vi "Receive Monitoring Frame.vi"(11 "Test Case In":refnum<class "Test HSU MCU V2.lvclass">) -> (0 "error out":errorcluster, 3 "Test Case Out":refnum<class "Test HSU MCU V2.lvclass">)   [LabVIEW 2024, in "Test HSU MCU V2.lvclass"]
uses:
  Test HSU MCU V2.lvclass
  C:/Program Files/National Instruments/LabVIEW 2024/vi.lib/Astemes/LUnit/Test Case.lvclass
  HSU MCU V2 CFG/HSU MCU V2 CFG.lvclass
  D:/git/HAL/HAL/Configurations/CFG JSON/CFG JSON.lvclass
  <vilib>/Astemes/LUnit/Test Case.lvclass/Test Case.ctl
  <vilib>/Astemes/LUnit/Append Pass Result.vi
  <vilib>/Astemes/LUnit/Append Fail Result.vi
  <vilib>/Astemes/LUnit/Run In UI.vi
  <vilib>/Utility/error.llb/Clear Errors.vi
  <vilib>/Astemes/LUnit/Test Case.lvclass
  Configurations/CFG JSON/CFG JSON.lvclass
panel:
  out "Output":variant
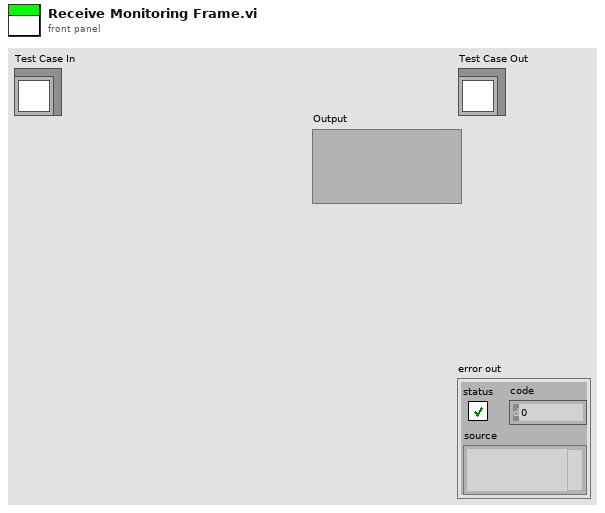
[diagram p1: front panel]
types:
  T1 = cluster{"Action":enum16{"Read", "Write"}, "Point Ident":string, "Data":variant}
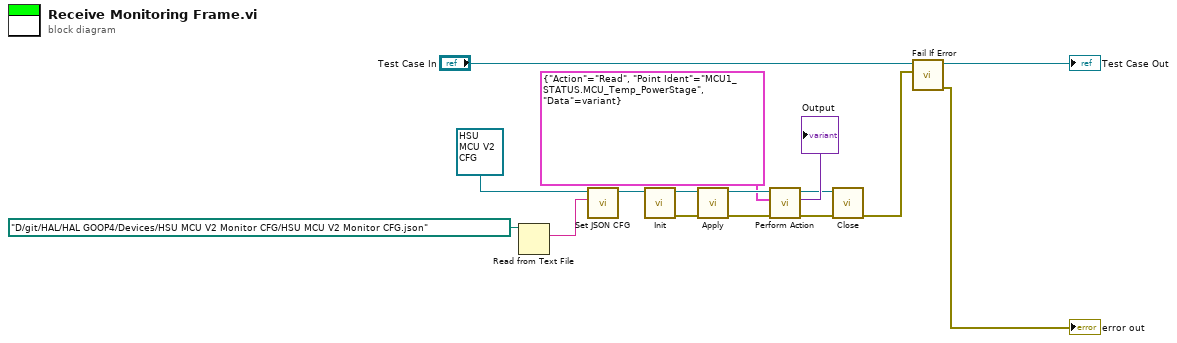
[diagram p0: block diagram]
diagram:
  n1 = Read from Text File(file (use dialog)=path "D:/git/HAL/HAL GOOP4/Devices/HSU MCU V2 Monitor CFG/HSU MCU V2 Monitor CFG.json") -> (text=w4:string)  [unwired: 3 in, 3 out]
  n2 = call "Set JSON CFG.vi"("<JSON> CFG"=w4, "CFG JSON in"=refnum<class "HSU MCU V2 CFG.lvclass"> refnum ("CFG Base in")) -> ("CFG JSON out"=w12:refnum<class "HSU MCU V2 CFG.lvclass">)  [unwired: 9 in]
  n3 = call-dynamic "Init.vi"("CFG Base in"=w12) -> ("error out"=w11:errorcluster, "CFG Base out"=w10:refnum<class "HSU MCU V2 CFG.lvclass">)  [unwired: 9 in]
  n4 = call-dynamic "Apply.vi"("error in"=w11, "HSU MCU V2 in"=w10) -> ("error out"=w9:errorcluster, "HSU MCU V2 out"=w8:refnum<class "HSU MCU V2 CFG.lvclass">)  [unwired: 8 in]
  n5 = call-dynamic "Perform Action.vi"("error in"=w9, "Input"=T1 {"Action"=enum."Read", "Point Ident"="MCU1_STATUS.MCU_Temp_PowerStage", "Data"=variant}, "HSU MCU V2 in"=w8) -> ("error out"=w7:errorcluster, "Output"=→"Output":variant, "HSU MCU V2 out"=w2:refnum<class "HSU MCU V2 CFG.lvclass">)  [unwired: 6 in]
  n6 = call-dynamic "Close.vi"("error in"=w7, "HSU MCU V2 Monitor CFG in"=w2) -> ("error out"=w3:errorcluster)  [unwired: 8 in, 1 out]
  n7 = call <vilib>:"Fail If Error.vi"("Assert error"=w3, "LUnit Test Case In"="Test Case In") -> ("error out"=→"error out":errorcluster, "LUnit Test Case Out"=→"Test Case Out":refnum<class "Test HSU MCU V2.lvclass">)  [unwired: 8 in]
